vi "SVT Third-octave Analysis (N Ch).vi"(0 "scaled signals [EU]":waveform(dbl)[](array[waveform])=[{"t0"=timestamp(0 s since 1904-01-01), "dt"=1.0, "Y"=[]}], 1 "restart averaging (F)":bool, 2 "reset filter (F)":bool, 5 "frequency range":T7={"low band"=enum."20 Hz", "high band"=enum."20000 Hz"}, 9 "dB On (T)":bool=TRUE, 11 "error in (no error)":errorcluster, 12 "averaging type":T8(ring), 13 "exp avg settings":T1={" mode"=enum."Fast", "time constant [ms]"=125.0} {"time constant [ms]" format="%.2f"}, 14 "equal confidence level [dB]":dbl=125.0 format="%.2f") -> (3 "filter settled":bool, 4 "octave spectra":T6(array[cluster]) {"band power" format="%.2f"; "nominal frequencies [Hz]" format="%.2f"}, 6 "unit labels":string[](array[string]), 8 "total band powers":dbl[](array[numeric]) format="%.2f", 10 "octave info":T2[](array[typedef]) {"engineering units" items=["custom..."=0, "V"=1, "A"=21, "C"=30, "pC"=31, "s"=32, "-"=29, "Pa"=2, "N"=20, "g"=3, "m/s^2"=4, "m/s"=5, "m"=6, "mm/s"=12, "mm"=13, "micron/s"=14, "micron"=15, "in/s^2"=7, "in/s"=8, "in"=9, "mil/s"=10, "mil"=11, "rad/s^2"=16, "rad/s"=17, "rad"=18, "deg/s^2"=26, "deg/s"=27, "deg"=28, "RPM"=22, "cycle/s^2"=23, "Hz"=24, "cycle"=25, "strain"=19]; "dB reference" format="%.2e"; "weighting filter" items=["Linear", "A-weighting", "B-weighting", "C-weighting", "ITU-R 468-4", "Dolby", "CCITT", "C-message", "Wb", "Wc", "Wd", "We", "Wf", "Wh", "Wj", "Wk", "Wm", "AES17 20 kHz lowpass", "AES17 40 kHz lowpass", "AES17 20 kHz highpass", "AES17 40 kHz highpass"]}, 15 "error out":errorcluster)   [LabVIEW 2017, in "SoundVib_Octave_2014 standard.lvlib"]
doc: "Performs a third-octave analysis on <B>scaled signal [EU]</B> in accordance with the IEC 61260 standard. You can use this polymorphic VI to perform third-octave analysis on a single channel or on N channels. The data type you wire to the <B>scaled signal [EU]</B> input determines the polymorphic instance to use."
uses:
  <vilib>/addons/Sound and Vibration/svt_Octave/SoundVib_Octave_2014 standard.lvlib
  <vilib>/addons/_NISVFA/_Shared subVIs/Controls/svc_Octave Info.ctl
  <vilib>/addons/_NISVFA/_Shared subVIs/Controls/svc_Octave Standard.ctl
  <vilib>/addons/_NISVFA/_Shared subVIs/Controls/svc_Weighting Filter Text Ring.ctl
  <vilib>/addons/_NISVFA/_Shared subVIs/Controls/svc_Engineering Units Text Ring.ctl
panel:
  out "# samples to settle":u64
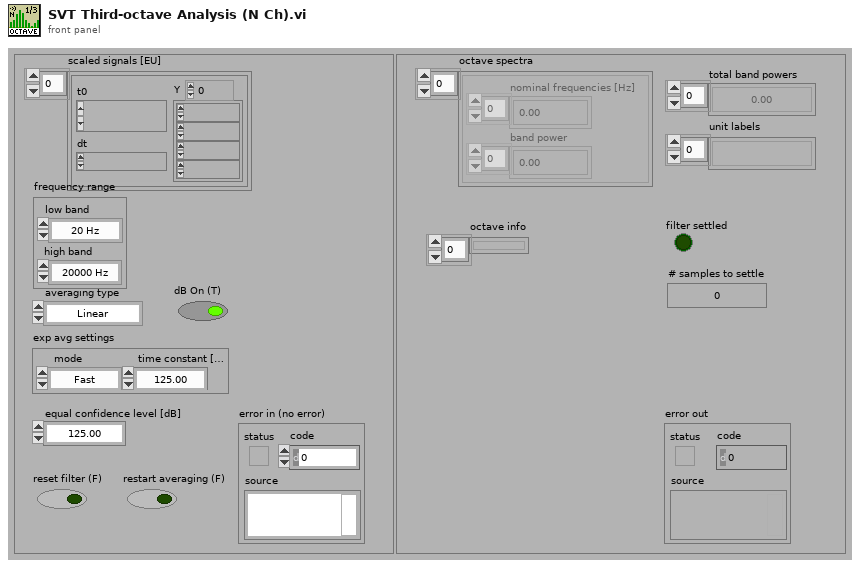
[diagram p1: front panel]
types:
  T1 = cluster{" mode":enum16{"Slow", "Fast", "Impulse", "Custom"}, "time constant [ms]":dbl}
  T2 = typedef "svc_Octave Info.ctl" = cluster{"standard":T3, "bandwidth":enum16{"1 octave", "1/3 octave", "1/6 octave", "1/12 octave", "1/24 octave"}, "low band":i32, "high band":i32, "weighting filter":T4, "dB reference":dbl, "dB On":bool, "unit label":string, "channel name":string, "description":string, "engineering units":T5, "custom label":string, "spectrum type":enum16{"power", "magnitude"}, "spectral density":bool, "filters settled":bool}
  T3 = typedef "svc_Octave Standard.ctl" = enum16{"ANSI S1.11", "IEC 61260"}
  T4 = typedef "svc_Weighting Filter Text Ring.ctl" = u16
  T5 = typedef "svc_Engineering Units Text Ring.ctl" = u16
  T6 = cluster{"nominal frequencies [Hz]":dbl[], "band power":dbl[]}[]
  T7 = cluster{"low band":enum16{"20 Hz", "25 Hz", "31.5 Hz", "40 Hz", "50 Hz", "63 Hz", "80 Hz", "100 Hz", "125 Hz", "160 Hz", "200 Hz", "250 Hz", "315 Hz", "400 Hz", "500 Hz", "630 Hz", "800 Hz", "1000 Hz", "1250 Hz", "1600 Hz", "2000 Hz", "2500 Hz", "3150 Hz", "4000 Hz", "5000 Hz", "6300 Hz", "8000 Hz", "10000 Hz", "12500 Hz", "16000 Hz", "20000 Hz"}, "high band":enum16{"20 Hz", "25 Hz", "31.5 Hz", "40 Hz", "50 Hz", "63 Hz", "80 Hz", "100 Hz", "125 Hz", "160 Hz", "200 Hz", "250 Hz", "315 Hz", "400 Hz", "500 Hz", "630 Hz", "800 Hz", "1000 Hz", "1250 Hz", "1600 Hz", "2000 Hz", "2500 Hz", "3150 Hz", "4000 Hz", "5000 Hz", "6300 Hz", "8000 Hz", "10000 Hz", "12500 Hz", "16000 Hz", "20000 Hz"}}
  T8 = enum16{"Linear", "Exponential", "Equal confidence", "Peak"}
  T9 = cluster{"standard":T3, "bandwidth":enum16{"1 octave", "1/3 octave", "1/6 octave", "1/12 octave", "1/24 octave"}}
  T10 = cluster{"dup nominal frequencies [Hz":dbl[], "band power [EU^2 rms]":dbl[]}[]
  T11 = cluster{"nominal frequencies [Hz]":dbl[], "band power [dB EU]":dbl[]}[]
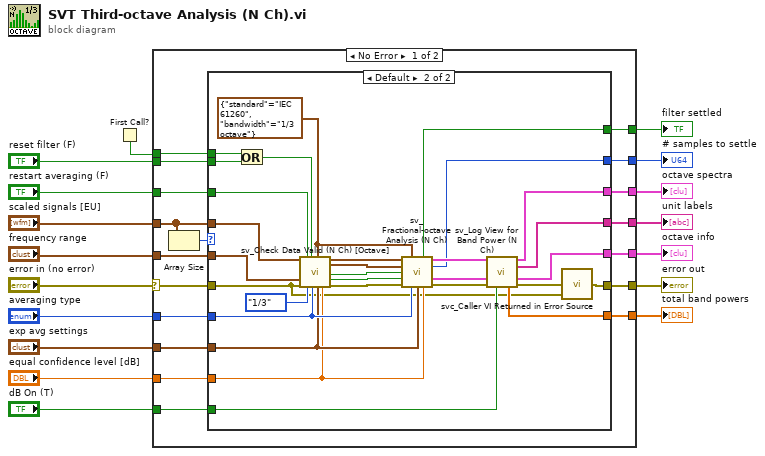
[diagram p0: block diagram]
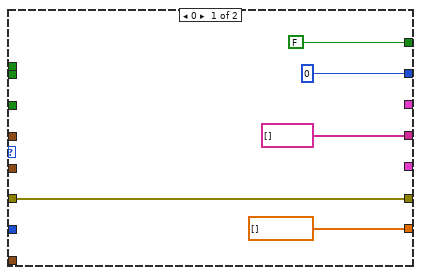
[diagram p2: hidden frame]
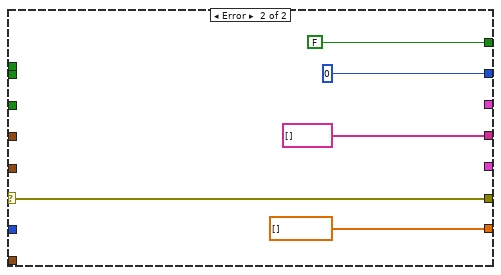
[diagram p3: hidden frame]
diagram:
  n1 = First Call?() -> (First Call?: T/F=w2:bool)
  n2 = case shown="No Error" "error in (no error)" {
    selector: "error in (no error)" -> [w25 w74]
    tunnel: "restart averaging (F)" -> [w35 _]
    tunnel: [w24 FALSE ("settled?")] -> w16
    tunnel: "dB On (T)" -> [w34 _]
    tunnel: "averaging type" -> [w33 _]
    tunnel: "frequency range" -> [w32 _]
    tunnel: "exp avg settings" -> [w31 _]
    tunnel: "equal confidence level [dB]" -> [w23 _]
    tunnel: [w30 dbl[] [] ("total band power(s) [dB EU]")] -> w10
    tunnel: "scaled signals [EU]" -> [w19 _]
    tunnel: [w26 w74] -> w8
    tunnel: [w29 _] -> w7
    tunnel: [w28 _] -> w6
    tunnel: [w27 string[] [] ("unit labels")] -> w5
    tunnel: "reset filter (F)" -> [w22 _]
    tunnel: w2 -> [w21 _]
    tunnel: [w20 u64 0 ("# samples to settle")] -> w1
    frame No Error {
      n3 = Array Size(array=w19) -> (size(s)=w18:i32)
      n4 = case shown="Default" w18 {
        tunnel: w35 -> [_ w69]
        tunnel: w34 -> [_ w64]
        tunnel: w33 -> [_ w62]
        tunnel: w32 -> [_ w61]
        tunnel: w31 -> [_ w60]
        tunnel: [dbl[] [] ("total band power(s) [dB EU]") w59] -> w30
        tunnel: [_ w56] -> w29
        tunnel: [_ w54] -> w28
        tunnel: [string[] [] ("unit labels") w53] -> w27
        tunnel: [w36 w52] -> w26
        tunnel: w25 -> [w36 w41]
        tunnel: [FALSE ("settled?") w48] -> w24
        tunnel: w23 -> [_ w47]
        tunnel: w22 -> [_ w46]
        tunnel: w21 -> [_ w45]
        tunnel: [u64 0 ("# samples to settle") w44] -> w20
        tunnel: w19 -> [_ w42]
        frame 0 {
        }
        frame Default {
          w43 = T9 {"standard"=enum."IEC 61260", "bandwidth"=enum."1/3 octave"} ("1/n Octave settings")
          n5 = Or(x=w45, y=w46) -> (x .or. y?=w50:bool)
          n6 = call <vilib>:"sv_Check Data Valid (N Ch) [Octave].vi"("Scaled signal(s)"=w42, "frequency range (1/3)"=w61, "error in (no error)"=w41, "restart averaging (F)"=w69, "bandwidth"=enum16{"1/1", "1/3", "1/n"}."1/3", "reset filter (F)"=w50, "averaging type"=w62, "1/n Octave settings"=w43, "exp avg settings"=w60, "equal confidence level [dB]"=w47) -> ("dup Scaled signal(s)"=w65:waveform(dbl)[], "band number"=w58:cluster{"low band":i32, "high band":i32}, "Restart averaging"=w67:bool, "Reset Filter"=w51:bool, "error out"=w68:errorcluster)  [unwired: 5 in]
          n7 = call <vilib>:"sv_Fractional-octave Analysis (N Ch).vi"("Scaled signal(s)"=w65, "1/n octave settings"=w43, "band number"=w58, "restart averaging (F)"=w67, "reset filter (F)"=w51, "error in (no error)"=w68, "averaging type"=w62, "exp avg settings"=w60, "equal confidence level [dB]"=w47) -> ("settled?"=w48:bool, "Octave measurements"=w63:T10, "# samples to settle"=w44:u64, "octave info"=w55:T2[], "error out"=w66:errorcluster)  [unwired: 2 in]
          n8 = call <vilib>:"sv_Log View for Band Power (N Ch).vi"("Octave measurements"=w63, "octave info"=w55, "error in (no error)"=w66, "dB On (T)"=w64) -> ("octave spectra"=w54:T11, "unit labels"=w53:string[], "octave info"=w56:T2[], "total band power(s) [dB EU]"=w59:dbl[], "error out"=w57:errorcluster)  [unwired: 7 in]
          n9 = call <vilib>:"svc_Caller VI Returned in Error Source.vi"("warning input to caller"=w41, "error in (no error)"=w57) -> ("error out"=w52:errorcluster)  [unwired: 3 in]
        }
      }
    }
    frame Error {
    }
  }
  "filter settled" <- w16
  "unit labels" <- w5
  "total band powers" <- w10
  "error out" <- w8
  "octave spectra" <- w6
  "octave info" <- w7
  "# samples to settle" <- w1
